vi "Set Button Pressed.vi"(8 "error in (no error)":errorcluster, 10 "Button Pressed?":bool, 11 "Button in":refnum<class "Button.lvclass">) -> (0 "error out":errorcluster, 3 "Button out":refnum<class "Button.lvclass">)   [LabVIEW 2018, in "Button.lvclass"]
uses:
  Button.lvclass
  Button.lvclass/Button.ctl
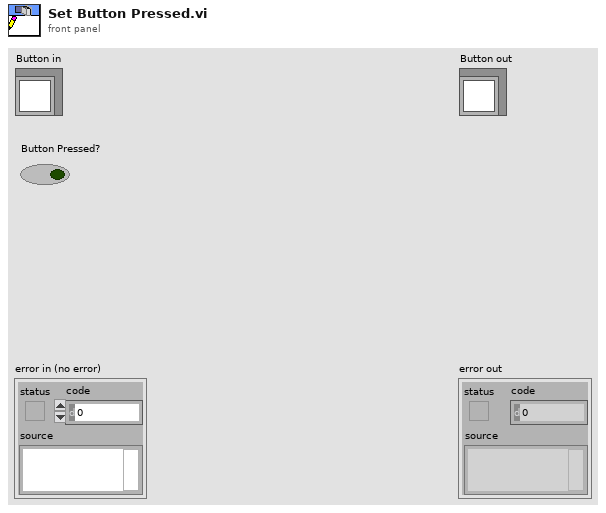
[diagram p1: front panel]
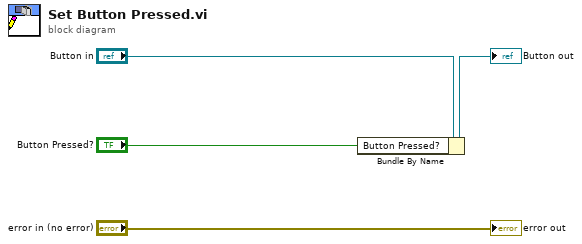
[diagram p0: block diagram]
diagram:
  n1 = Bundle By Name(cluster="Button in", "Button Pressed?"="Button Pressed?") -> (→"Button out":refnum<class "Button.lvclass">)
  "error out" <- "error in (no error)"
